vi "Gauss.vi"(0 "x":dbl[](array[numeric]), 5 "a1":dbl, 7 "a2":dbl, 9 "a3":dbl, 11 "a4":dbl) -> (4 "x+y":dbl[](array[numeric]))   [LabVIEW 2015]
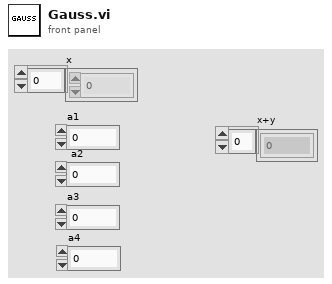
[diagram p1: front panel]
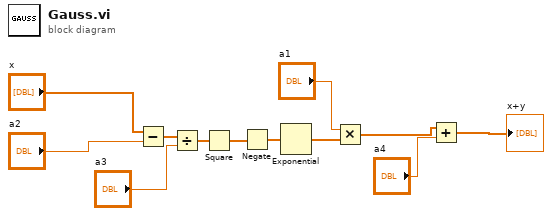
[diagram p0: block diagram]
diagram:
  n1 = Subtract(x="x", y="a2") -> (x-y=w9:dbl[])
  n2 = Divide(x=w9, y="a3") -> (x/y=w8:dbl[])
  n3 = Square(x=w8) -> (x^2=w11:dbl[])
  n4 = Negate(x=w11) -> (-x=w10:dbl[])
  n5 = Exponential(1:w10) -> (0:w12:dbl[])
  n6 = Multiply(x="a1", y=w12) -> (x*y=w7:dbl[])
  n7 = Add(x=w7, y="a4") -> (x+y=→"x+y":dbl[])
